vi "FinalLinearStage.vi"() -> ()   [LabVIEW 2016]
uses:
  <vilib>/Instr/_visa.llb/VISA Configure Serial Port (Instr).vi
panel:
  in  "Wait Time (ms)":u32
  in  "Change in Distance (mm)":dbl
  in  "Total Distance (mm)":dbl
  in  "Starting Distance (mm)":dbl
  in  "Extra Commands":string
  out "Response":string
  in  "Read":bool
  in  "Stop":bool
  in  "Start":bool
  # "** Total distance must be less than 200mm"
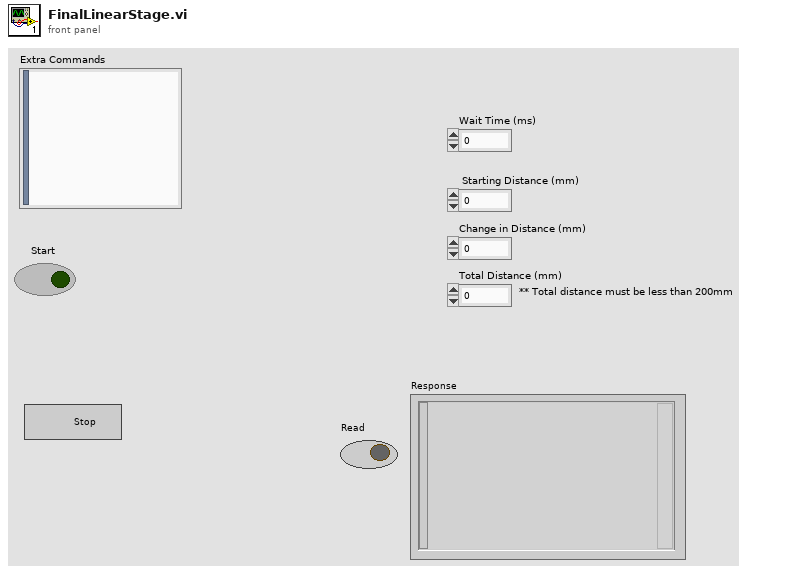
[diagram p1: front panel]
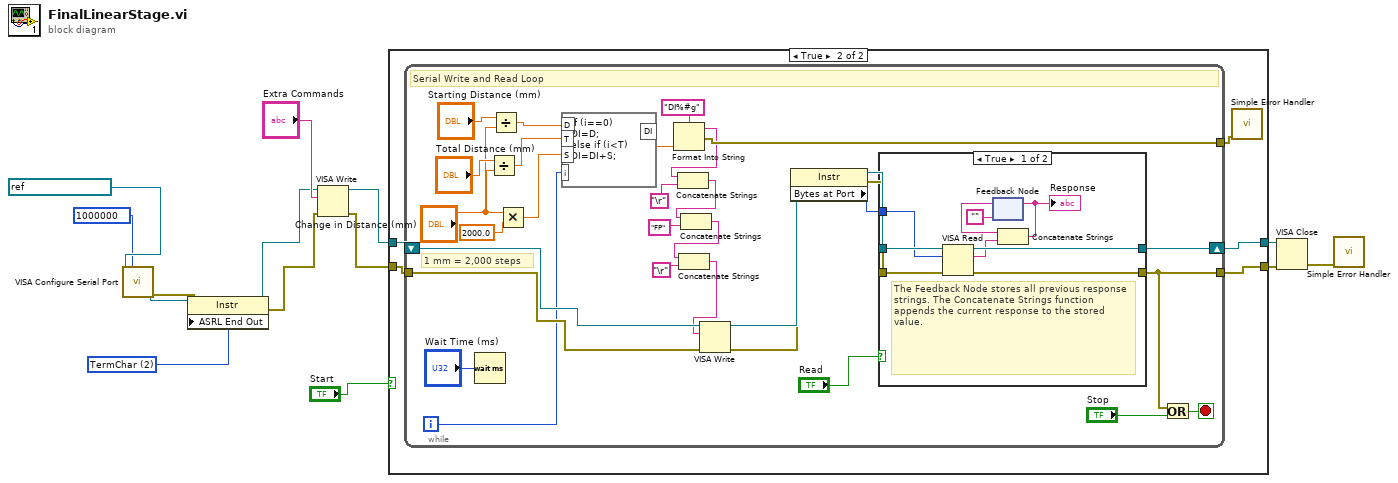
[diagram p0: block diagram]
diagram:
  w11 = u16 2 items=["None", "Last Bit", "TermChar", "Break"] ("Serial Settings:End Mode for Writes")
  n1 = call-poly "VISA Configure Serial Port"("VISA resource name"=refnum<visa-resource-name> "ASRL1::INSTR", "timeout (10sec)"=u32 1000000) -> ("VISA resource name out"=w13:refnum<visa-resource-name>, "error out"=w12:errorcluster)  [unwired: 12 in]
  n2 = property class="Instr"(reference=w13, error in=w12, "ASRL End Out"=w11) -> (reference out=w5:refnum<visa-resource-name>, error out=w4:errorcluster)
  n3 = VISA Write(VISA resource name=w5, write buffer="Extra Commands", error in (no error)=w4) -> (VISA resource name out=w2:refnum<visa-resource-name>, error out=w3:errorcluster)  [unwired: 1 out]
  n4 = case shown="True" "Start" {
    tunnel: [w16 w21] -> w8
    tunnel: [w15 w20] -> w7
    tunnel: w3 -> [w16 w19]
    tunnel: w2 -> [w15 w18]
    frame False {
    }
    frame True {
      n5 = while {
        shift-right: [w52] -> w20
        shift-left: w18 -> [w43]
        tunnel: w19 -> [w51]
        tunnel: [w30] -> w21
        tunnel: [w29] -> w17
        i -> [w42]
        stop <- w49 stop-if-true
        # "1 mm = 2,000 steps"
        # "Serial Write and Read Loop"
        n6 = Wait (ms)(milliseconds to wait="Wait Time (ms)") -> ()  [unwired: 1 out]
        n7 = Divide(x="Total Distance (mm)", y="Change in Distance (mm)") -> (x/y=w36:dbl)
        n8 = Divide(x="Starting Distance (mm)", y="Change in Distance (mm)") -> (x/y=w41:dbl)
        n9 = Multiply(x="Change in Distance (mm)", y=2000.0) -> (x*y=w37:dbl)
        n10 = formula code="if (i==0)\nDI=D;\nelse if (i<T)\nDI=DI+S;"("D"=w41, "T"=w36, "S"=w37, "i"=w42) -> ("DI"=w33:dbl)
        n11 = Format Into String(format string="DI%#g", w33) -> (resulting string=w28:string, error out=w29:errorcluster)  [unwired: 2 in]
        n12 = Concatenate Strings(w28, "\r") -> (w27:string)
        n13 = Concatenate Strings(w27, "FP" ("string")) -> (w26:string)
        n14 = Concatenate Strings(w26, "\r") -> (w25:string)
        n15 = VISA Write(VISA resource name=w43, write buffer=w25, error in (no error)=w51) -> (VISA resource name out=w46:refnum<visa-resource-name>, error out=w31:errorcluster)  [unwired: 1 out]
        n16 = property class="Instr"(reference=w46, error in=w31) -> (reference out=w45:refnum<visa-resource-name>, error out=w44:errorcluster, "Bytes at Port"=w47:u32)
        n17 = case shown="True" "Read" {
          tunnel: [w59 w63] -> w52
          tunnel: w45 -> [w61 w63]
          tunnel: [w58 w62] -> w30
          tunnel: w44 -> [w60 w62]
          tunnel: w47 -> [w53 _]
          frame True {
            # "The Feedback Node stores all previous response strings. The Concatenate Strings function appends the current response to the stored value."
            n18 = VISA Read(VISA resource name=w61, byte count=w53, error in (no error)=w60) -> (VISA resource name out=w59:refnum<visa-resource-name>, read buffer=w57:string, error out=w58:errorcluster)  [unwired: 1 out]
            n19 = feedback #1("") -> (w56:string)
            n20 = Concatenate Strings(w56, w57) -> (w55:string)
            "Response" <- w55
            n21 = feedback-in #1(w55) -> ()
          }
          frame False {
          }
        }
        n22 = Or(x=w30, y="Stop") -> (x .or. y?=w49:bool)
      }
      n23 = call <vilib>:"Simple Error Handler.vi"("error in (no error)"=w17) -> ()  [unwired: 1 in, 8 out]
    }
  }
  n24 = VISA Close(VISA resource name=w7, error in (no error)=w8) -> (error out=w9:errorcluster)
  n25 = call <vilib>:"Simple Error Handler.vi"("error in (no error)"=w9) -> ()  [unwired: 1 in, 8 out]
